vi "Initialize-Shutdown.vi"(8 "Error In":errorcluster) -> (0 "Error Out":errorcluster)   [LabVIEW 2018, in "Tests.lvlib" / "SSH.lvlib"]
uses:
  SSH.lvlib
  <vilib>/addons/_JKI Toolkits/Caraya/classes/Test/Test.lvclass
  <vilib>/addons/_JKI Toolkits/Caraya/classes/Assert/Assert.lvclass
  src/Toolkit/SSH/SSH.lvclass
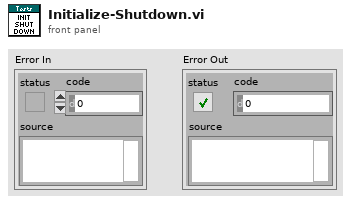
[diagram p1: front panel]
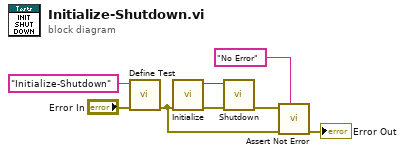
[diagram p0: block diagram]
diagram:
  n1 = call <vilib>:"Define Test.vi"("error in (no error)"="Error In", "Label (VI Title)"="Initialize-Shutdown") -> ("error out"=w4:errorcluster)  [unwired: 9 in]
  n2 = call "Initialize.vi"("Error In"=w4) -> ("Error Out"=w3:errorcluster, "SSH"=w1:refnum<class "SSH.lvclass">)  [unwired: 9 in]
  n3 = call "Shutdown.vi"("Error In"=w3, "SSH"=w1) -> ("Error Out"=w2:errorcluster)  [unwired: 9 in]
  n4 = call <vilib>:"Assert Not Error.vi"("Label"="No Error", "error in (no error)"=w4, "Not Error?"=w2) -> ("error out"=→"Error Out":errorcluster)  [unwired: 8 in]
